vi "is valid.vi"(11 "connection in":refnum<class "Queue connection.lvclass">) -> (3 "valid":bool)   [LabVIEW 2015, in "Queue connection.lvclass"]
uses:
  Queue connection.lvclass
  Queue connection.lvclass/Queue connection.ctl
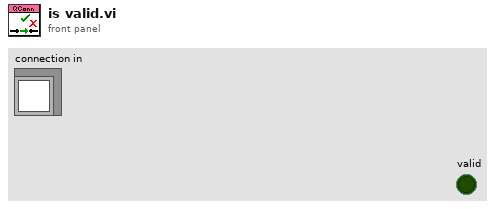
[diagram p1: front panel]
types:
  T1 = typedef "Queue connection.lvclass/queue pair.ctl" = cluster{"to pair":refnum<queue>, "from pair":refnum<queue>}
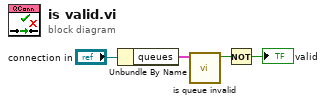
[diagram p0: block diagram]
diagram:
  n1 = Unbundle By Name("connection in") -> ("queues"=w3:T1)
  n2 = call "is queue invalid.vi"("queues"=w3) -> ("queue invalid?"=w2:bool)  [unwired: 10 in]
  n3 = Not(x=w2) -> (.not. x?=→"valid":bool)
